vi "Simple DAQ.vi"() -> ()   [LabVIEW 2014]
uses:
  Classes/DAQ/DAQ Parameters.ctl
  Classes/DAQ/Trigger Source.ctl
  Classes/DAQ/Trigger Slope.ctl
  Type Defs/OCT DAQ Channel Data Type.ctl
  Classes/DAQ/Clock Control.ctl
  Simple DAQ States.ctl
  Classes/DAQ Control Functional Global States.ctl
  Classes/DAQ/ATS660/ATS660 Class.lvclass
  Classes/DAQ/ATS9462/ATS9462 Class.lvclass
  Classes/DAQ/ATS9350/ATS9350.lvclass
  Classes/Laser/Insite/Insight.lvclass
  <vilib>/Analysis/4window.llb/Hanning Window (DBL).vi
  <vilib>/Analysis/2dsp.llb/Real FFT.vi
  <vilib>/Analysis/4window.llb/AllCosWindow (DBL).vi
  Classes/DAQ/DAQ Class.lvclass
  <vilib>/Analysis/NI_AALPro.lvlib
panel:
  out "Path append":string="\\Insight LASER\\"
  in  "Record Data":bool
  in  "LASER Source":enum16{"INSIGHT", "SANTEC"}(ring)
  out "offset":dbl format="%.2f"
  out "mult":dbl
  in  "FFT Display":bool
  out "Frequency Domain":dbl[][](graph)
  in  "Pause Button":bool
  in  "Stop Button":bool
  in  "Play Button":bool
  out "Time Domain":dbl[][](graph)
  in  "DAQ Parameters Out":T1={"Points Per A-Scan"=1024, "A-Scans Per B-Scan"=250, "Number of B-Scans"=1, "A-Scans Per Transfer"=250, "Trigger Voltage"=200.0, "Trigger Source"=enum."External", "Trigger Slope"=enum."Rising", "Channel"=enum."Channel 1", "Clock"=enum."External Clock", "Bits per Sample"=16.0, "Range"=2.0}
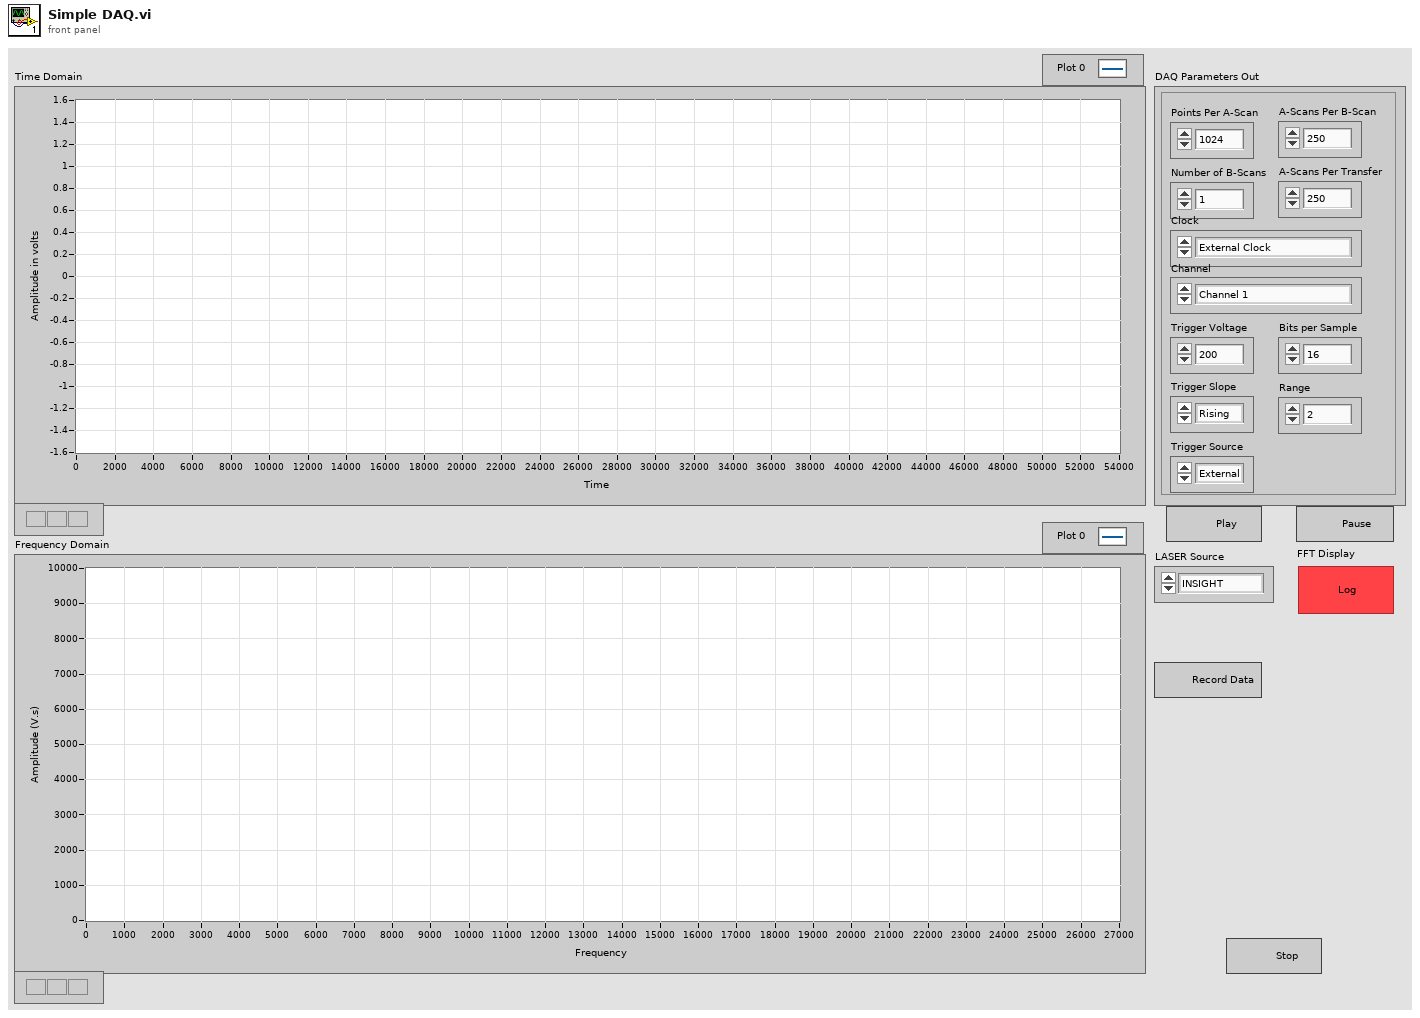
[diagram p1: front panel]
types:
  T1 = typedef "DAQ Class.lvclass/DAQ Parameters.ctl" = cluster{"Points Per A-Scan":u32, "A-Scans Per B-Scan":u32, "Number of B-Scans":u32, "A-Scans Per Transfer":u32, "Trigger Voltage":sgl, "Trigger Source":T2, "Trigger Slope":T3, "Channel":T4, "Clock":T5, "Bits per Sample":dbl, "Range":dbl}
  T2 = typedef "DAQ Class.lvclass/Trigger Source.ctl" = enum16{"External", "Channel A", "Channel B"}
  T3 = typedef "DAQ Class.lvclass/Trigger Slope.ctl" = enum16{"Rising", "Falling"}
  T4 = typedef "OCT DAQ Channel Data Type.ctl" = enum16{"Channel 1", "Channel 2", "Channel 1 and 2"}
  T5 = typedef "DAQ Class.lvclass/Clock Control.ctl" = enum16{"Internal Clock", "External Clock"}
  T6 = typedef "Simple DAQ States.ctl" = enum16{"Initialize DAQ", "Reset DAQ", "Configure DAQ", "Acquire", "Acquire and Save", "Stop"}
  T7 = typedef "DAQ Control Functional Global States.ctl" = enum16{"Status", "Set Processing Finished", "Reset", "Clear", "Set DAQ Finished"}
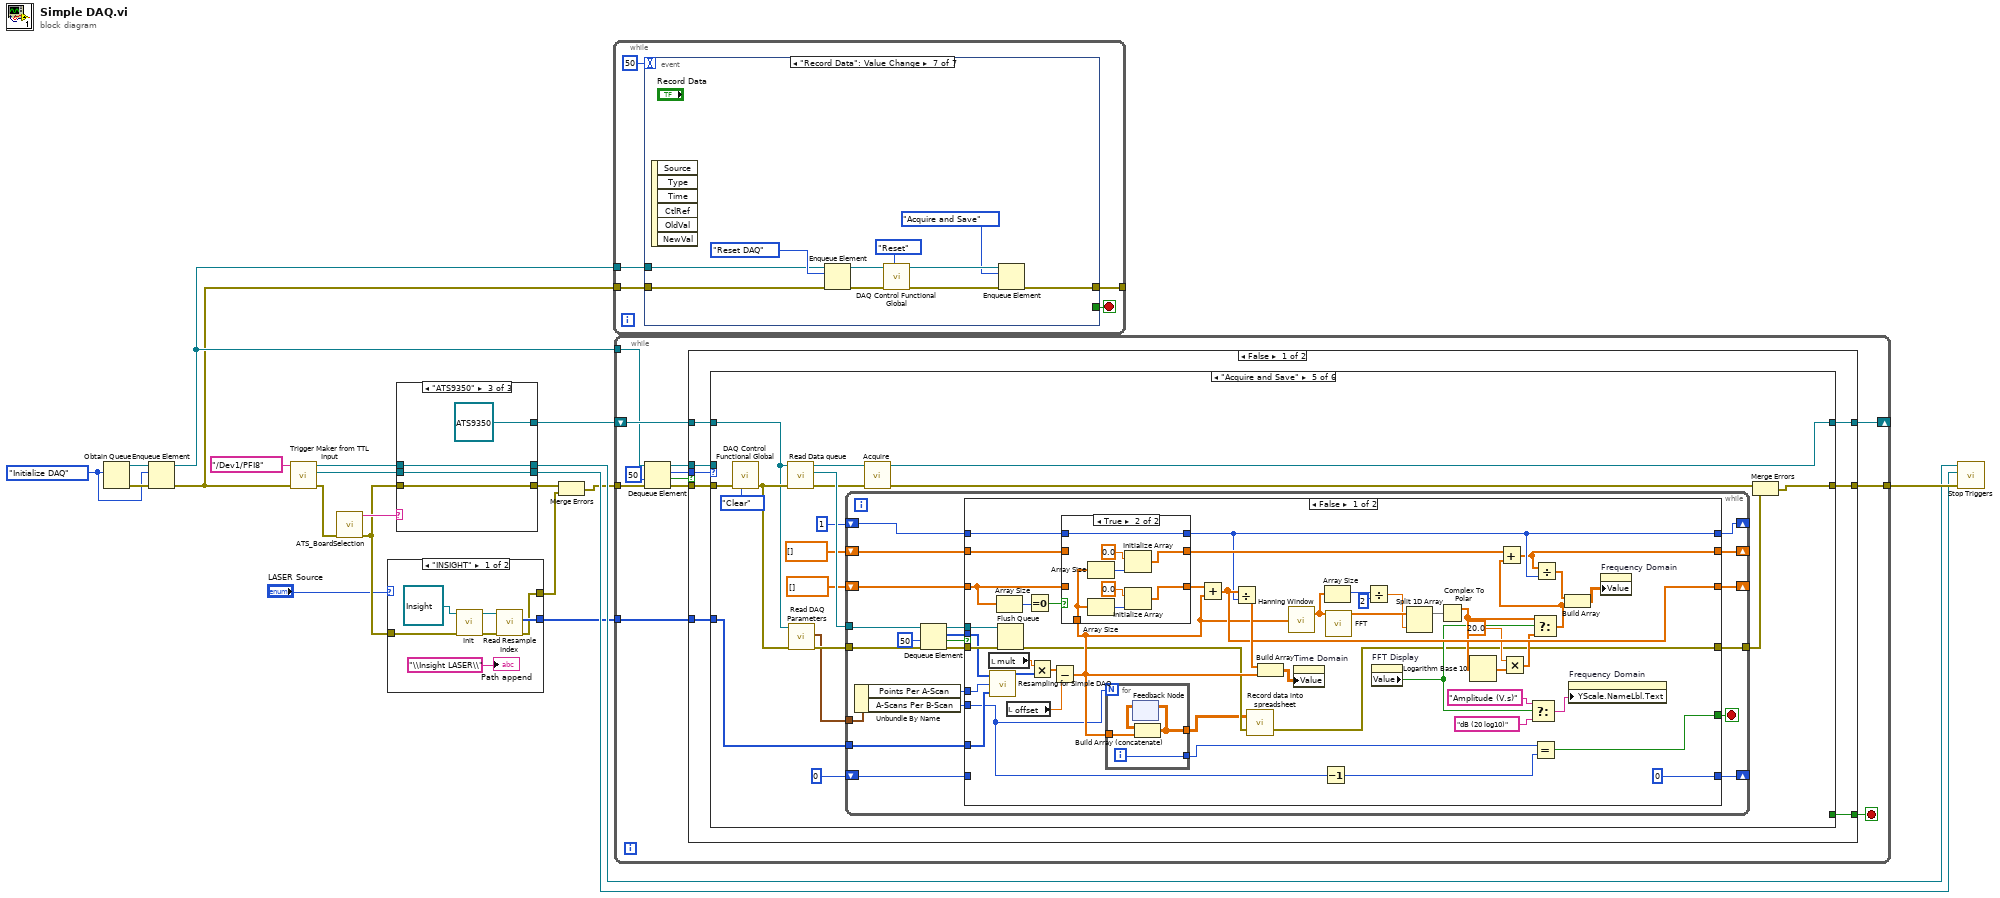
[diagram p0: block diagram]
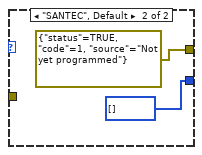
[diagram p2: hidden frame]
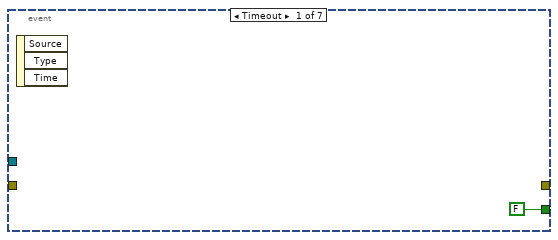
[diagram p3: hidden frame]
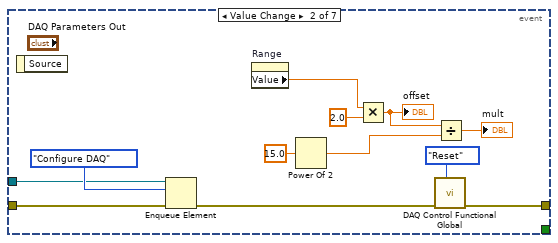
[diagram p4: hidden frame]
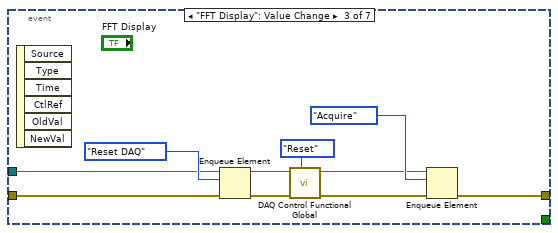
[diagram p5: hidden frame]
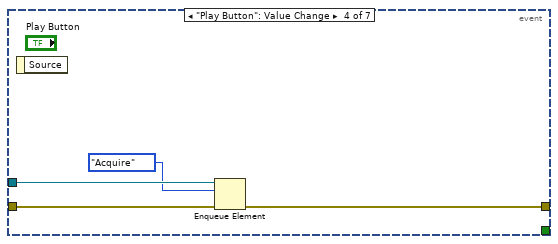
[diagram p6: hidden frame]
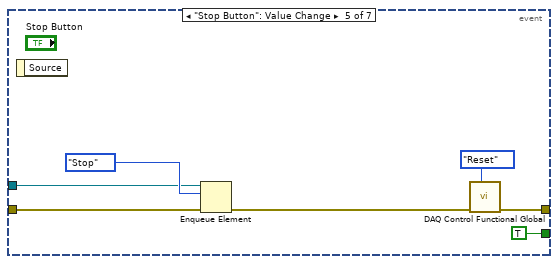
[diagram p7: hidden frame]
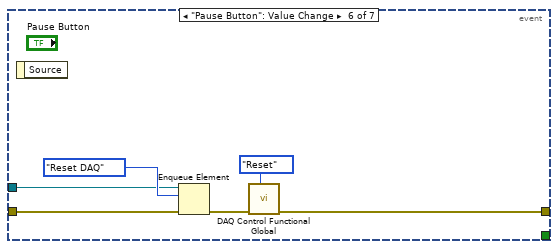
[diagram p8: hidden frame]
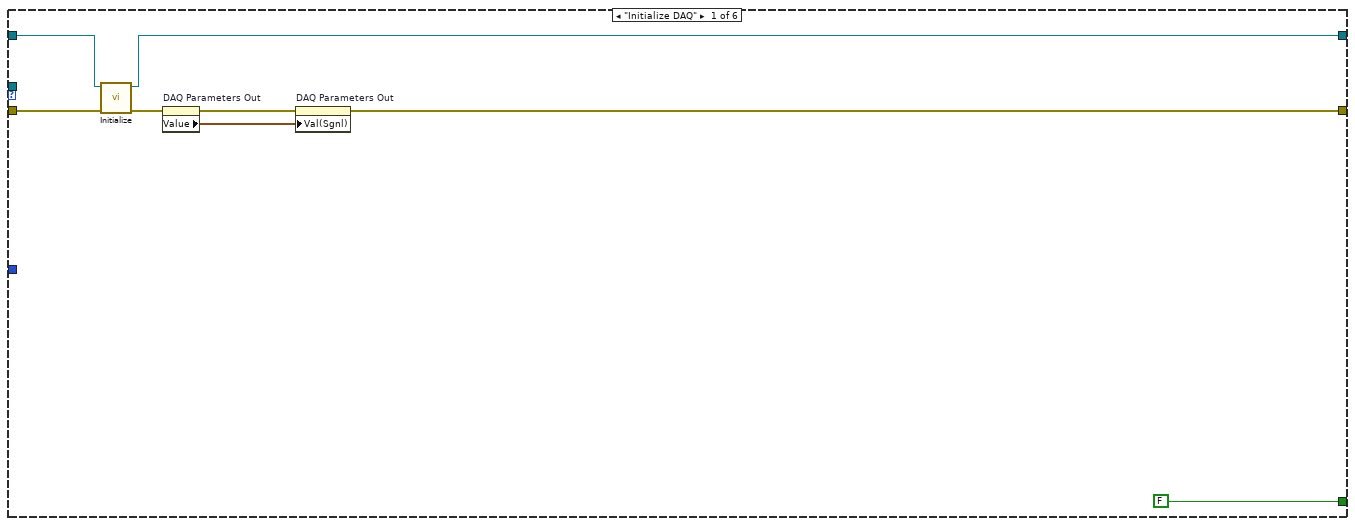
[diagram p9: hidden frame]
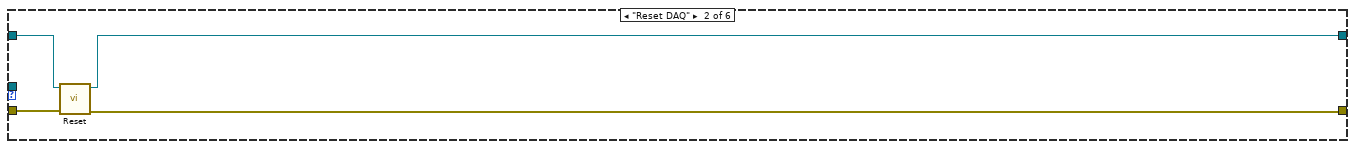
[diagram p10: hidden frame]
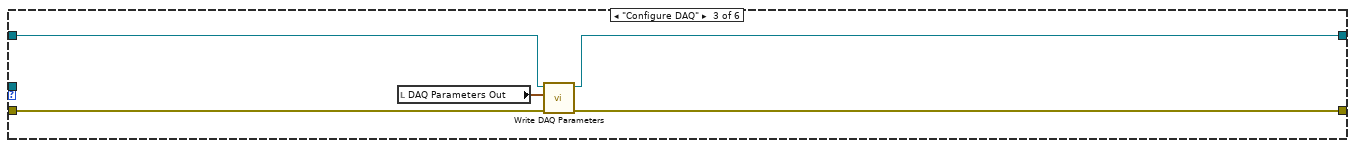
[diagram p11: hidden frame]
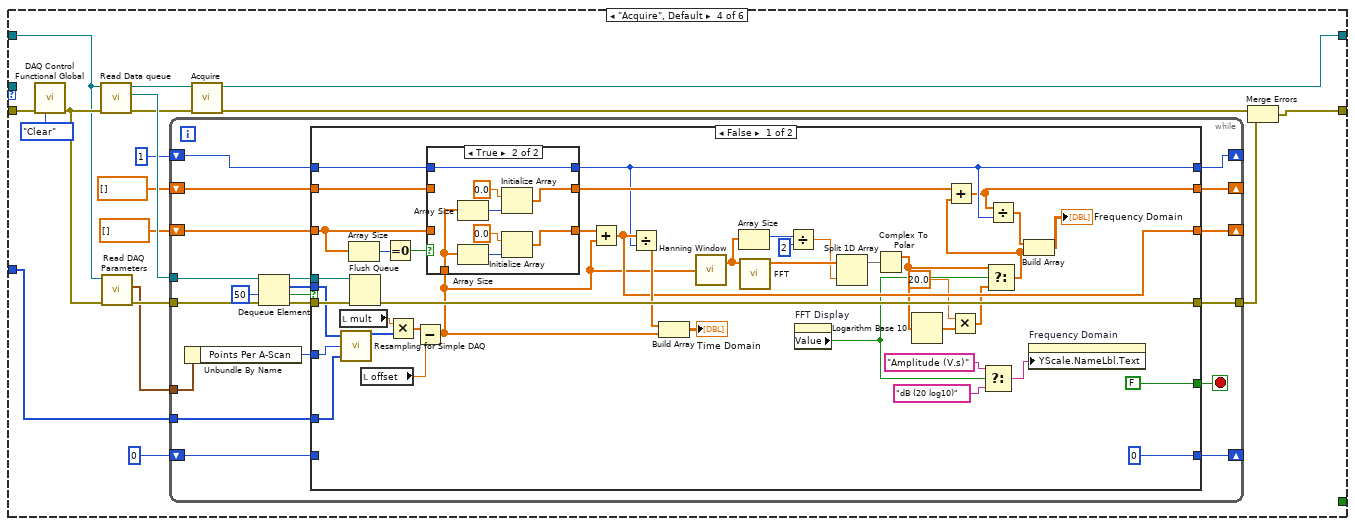
[diagram p12: hidden frame]
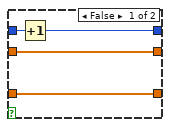
[diagram p13: hidden frame]
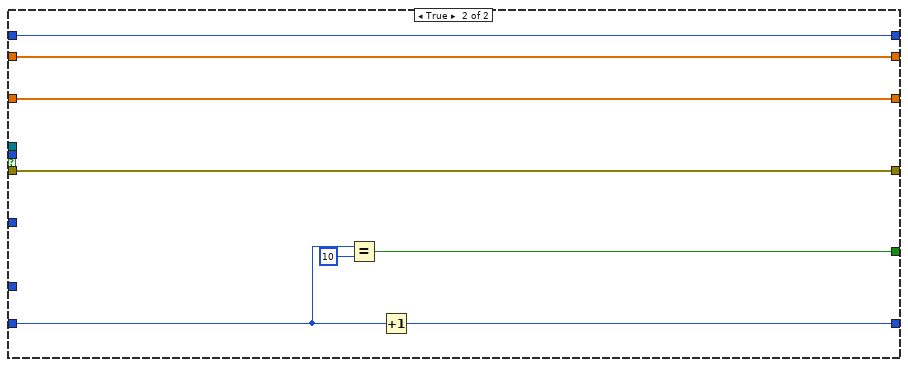
[diagram p14: hidden frame]
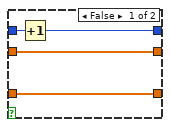
[diagram p15: hidden frame]
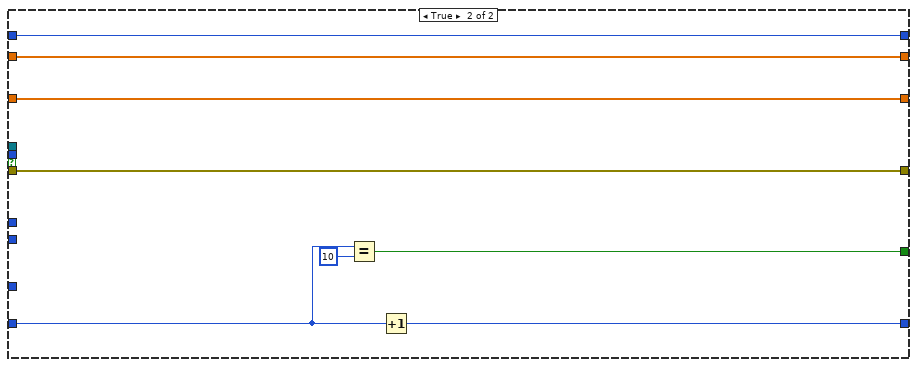
[diagram p16: hidden frame]
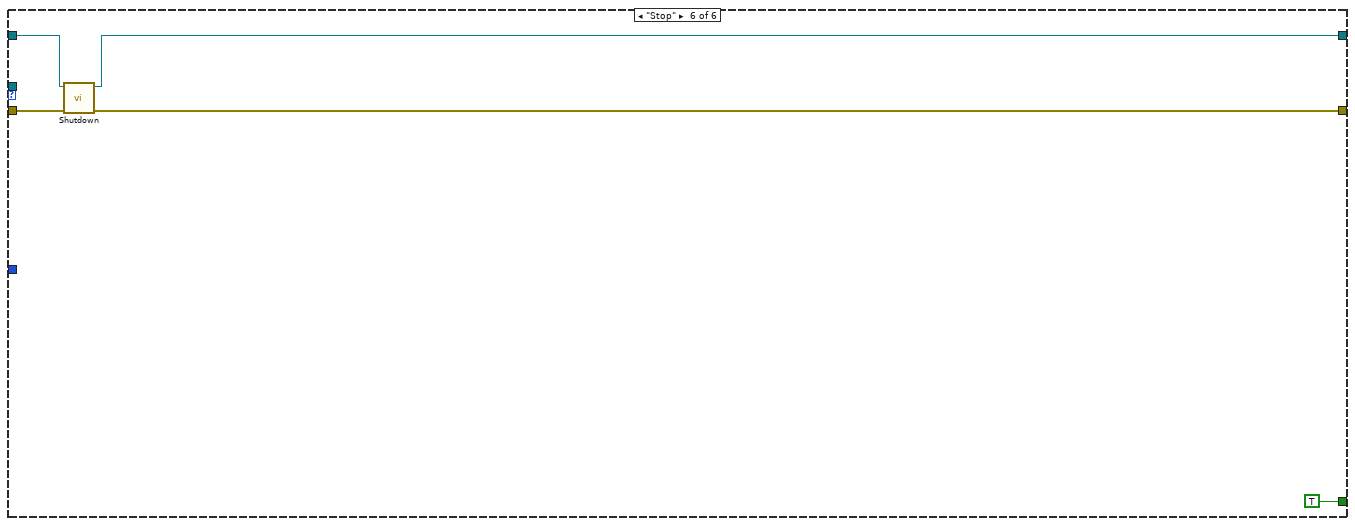
[diagram p17: hidden frame]
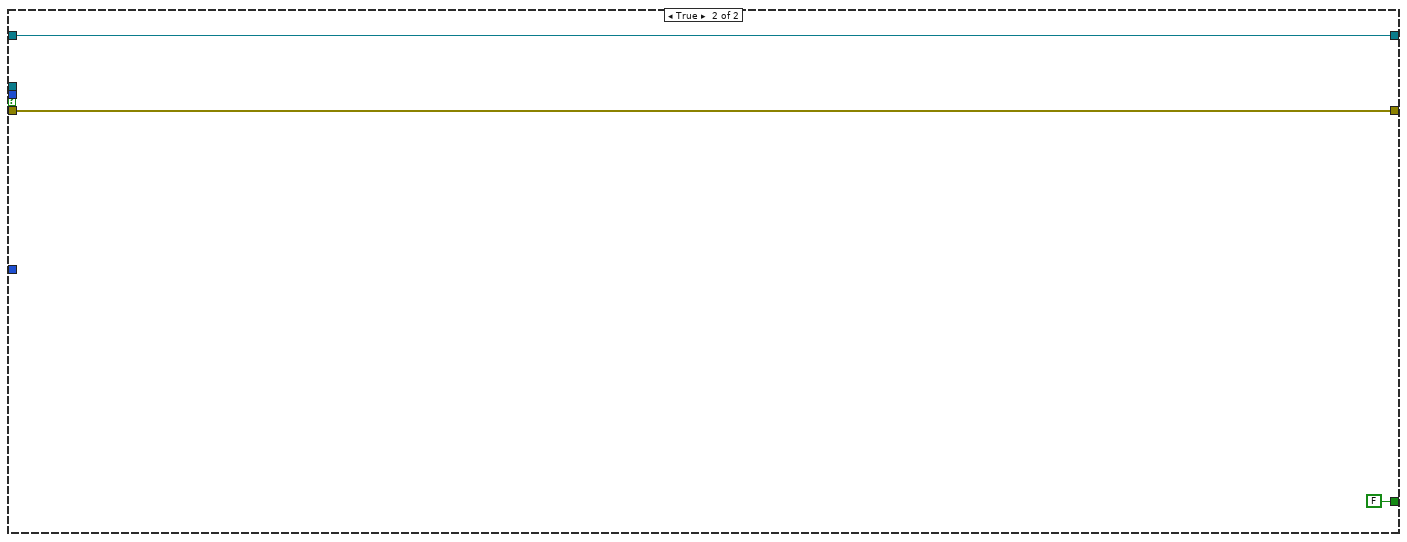
[diagram p18: hidden frame]
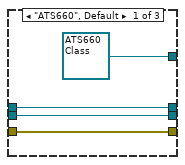
[diagram p19: hidden frame]
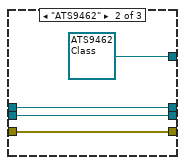
[diagram p20: hidden frame]
diagram:
  w8 = Simple_DAQ_States."Initialize DAQ" ("Simple OCT States")
  n1 = Obtain Queue(element data type=w8) -> (queue out=w12:refnum<queue>, error out=w11:errorcluster)  [unwired: 4 in, 1 out]
  n2 = Enqueue Element(queue=w12, element=w8, error in (no error)=w11) -> (queue out=w10:refnum<queue>, error out=w9:errorcluster)  [unwired: 1 in, 1 out]
  n3 = call "Trigger Maker from TTL Input.vi"("Error in"=w9, "Master Trigger In from Laser (TTL)"=tag "/Dev1/PFI8") -> ("error out"=w7:errorcluster, "Alazar Task"=w18:refnum<k21>, "AFG11000 Task"=w19:refnum<k21>)  [unwired: 7 in]
  n4 = call "ATS_BoardSelection.vi"("error in (no error)"=w7) -> ("error out"=w5:errorcluster, "Board"=w6:string)  [unwired: 9 in]
  n5 = case shown="\"INSIGHT\"" "LASER Source" {
    tunnel: w5 -> [w21 _]
    tunnel: [w27 u32[] [] ("Resample Index")] -> w3
    tunnel: [w26 errorcluster {"status"=TRUE, "code"=1, "source"="Not yet programmed"} ("error constant")] -> w1
    frame "INSIGHT" {
      n6 = call-dynamic "Init.vi"("error in (no error)"=w21, "Insite in"=refnum<class "Insight.lvclass"> refnum ("Insight.lvclass")) -> ("error out"=w22:errorcluster, "Insite out"=w23:refnum<class "Insight.lvclass">)  [unwired: 8 in]
      n7 = call-dynamic "Read Resample Index.vi"("error in (no error)"=w22, "Laser in"=w23) -> ("error out"=w26:errorcluster, "Resample Index"=w27:u32[])  [unwired: 7 in, 1 out]
      "Path append" <- "\\Insight LASER\\"
    }
    frame "SANTEC", Default {
    }
  }
  n8 = case shown="\"ATS9350\"" w6 {
    tunnel: w5 -> [w31 w34 w39]
    tunnel: [w33 w36 w41] -> w14
    tunnel: w19 -> [w33 w36 w41]
    tunnel: w18 -> [w32 w35 w40]
    tunnel: [w32 w35 w40] -> w13
    tunnel: [w31 w34 w39] -> w17
    tunnel: [refnum<class "ATS660 Class.lvclass"> refnum ("ATS660 Class.lvclass") refnum<class "ATS9462 Class.lvclass"> refnum ("ATS9462 Class.lvclass") refnum<class "ATS9350.lvclass"> refnum ("ATS9350.lvclass")] -> w16
    frame "ATS660", Default {
    }
    frame "ATS9462" {
    }
    frame "ATS9350" {
    }
  }
  n9 = Merge Errors(w17, w1) -> (w2:errorcluster)
  n10 = while {
    tunnel: w10 -> [w43]
    tunnel: w9 -> [w44]
    tunnel: [w42] -> _
    stop <- w46 stop-if-true
    n11 = event shown="[6] \"Record Data\": Value Change" {
      selector: _ -> [_ _ _ _ _ _ _]
      dyn-events: _ -> [_ _ _ _ _ _ _]
      timeout: 50 -> [_ _ _ _ _ _ _]
      tunnel: [FALSE _ _ _ TRUE _ _] -> w46
      tunnel: w44 -> [_ w56 w64 w71 w74 w84 w87]
      tunnel: w43 -> [_ w57 w65 w72 w73 w83 w88]
      tunnel: [_ w54 w62 w70 w75 w80 w86] -> w42
      event Timeout {
        n12 = event-data() -> ()  [unwired: 1 in, 3 out]
      }
      event Value Change {
        n13 = event-data() -> ()  [unwired: 1 in, 1 out]
        n14 = Enqueue Element(queue=w57, element=Simple_DAQ_States."Configure DAQ" ("Simple OCT States"), error in (no error)=w56) -> (error out=w55:errorcluster)  [unwired: 1 in, 2 out]
        n15 = property on="Range" class="DigNum (strict)"() -> ("Value"=w49:dbl)  [unwired: 2 in, 2 out]
        n16 = Power Of 2(x=15.0) -> (2^x=w52:dbl)
        n17 = Multiply(x=w49, y=2.0 ("Offset")) -> (x*y=w48:dbl)
        "offset" <- w48
        n18 = call "DAQ Control Functional Global.vi"("State"=DAQ_Control_Functional_Global_States."Reset", "Error In"=w55) -> ("Error Out"=w54:errorcluster)  [unwired: 6 in, 3 out]
        n19 = Divide(x=w48, y=w52) -> (x/y=→"mult":dbl)
      }
      event "FFT Display": Value Change {
        n20 = event-data() -> ()  [unwired: 1 in, 6 out]
        n21 = Enqueue Element(queue=w65, element=Simple_DAQ_States."Reset DAQ" ("Simple OCT States"), error in (no error)=w64) -> (queue out=w60:refnum<queue>, error out=w68:errorcluster)  [unwired: 1 in, 1 out]
        n22 = call "DAQ Control Functional Global.vi"("State"=DAQ_Control_Functional_Global_States."Reset", "Error In"=w68) -> ("Error Out"=w61:errorcluster)  [unwired: 6 in, 3 out]
        n23 = Enqueue Element(queue=w60, element=Simple_DAQ_States."Acquire" ("Simple OCT States"), error in (no error)=w61) -> (error out=w62:errorcluster)  [unwired: 1 in, 2 out]
      }
      event "Play Button": Value Change {
        n24 = event-data() -> ()  [unwired: 1 in, 1 out]
        n25 = Enqueue Element(queue=w72, element=Simple_DAQ_States."Acquire" ("Simple OCT States"), error in (no error)=w71) -> (error out=w70:errorcluster)  [unwired: 1 in, 2 out]
      }
      event "Stop Button": Value Change {
        n26 = event-data() -> ()  [unwired: 1 in, 1 out]
        n27 = Enqueue Element(queue=w73, element=Simple_DAQ_States."Stop" ("Simple OCT States"), error in (no error)=w74) -> (error out=w76:errorcluster)  [unwired: 1 in, 2 out]
        n28 = call "DAQ Control Functional Global.vi"("State"=DAQ_Control_Functional_Global_States."Reset", "Error In"=w76) -> ("Error Out"=w75:errorcluster)  [unwired: 6 in, 3 out]
      }
      event "Pause Button": Value Change {
        n29 = event-data() -> ()  [unwired: 1 in, 1 out]
        n30 = Enqueue Element(queue=w83, element=Simple_DAQ_States."Reset DAQ" ("Simple OCT States"), error in (no error)=w84) -> (error out=w81:errorcluster)  [unwired: 1 in, 2 out]
        n31 = call "DAQ Control Functional Global.vi"("State"=DAQ_Control_Functional_Global_States."Reset", "Error In"=w81) -> ("Error Out"=w80:errorcluster)  [unwired: 6 in, 3 out]
      }
      event "Record Data": Value Change {
        n32 = event-data() -> ()  [unwired: 1 in, 6 out]
        n33 = Enqueue Element(queue=w88, element=Simple_DAQ_States."Reset DAQ" ("Simple OCT States"), error in (no error)=w87) -> (queue out=w94:refnum<queue>, error out=w89:errorcluster)  [unwired: 1 in, 1 out]
        n34 = call "DAQ Control Functional Global.vi"("State"=DAQ_Control_Functional_Global_States."Reset", "Error In"=w89) -> ("Error Out"=w93:errorcluster)  [unwired: 6 in, 3 out]
        n35 = Enqueue Element(queue=w94, element=Simple_DAQ_States."Acquire and Save" ("Simple OCT States"), error in (no error)=w93) -> (error out=w86:errorcluster)  [unwired: 1 in, 2 out]
      }
    }
  }
  n36 = while {
    tunnel: w2 -> [w104]
    tunnel: w10 -> [w100]
    tunnel: [w97] -> w15
    shift-right: [w96] -> _
    shift-left: w16 -> [w106]
    tunnel: w3 -> [w95]
    stop <- w105 stop-if-true
    n37 = Dequeue Element(queue=w100, timeout in ms (-1)=50, error in (no error)=w104) -> (queue out=w99:refnum<queue>, element=w98:T6, timed out?=w101:bool, error out=w103:errorcluster)
    n38 = case shown="False" w101 {
      tunnel: w103 -> [w114 w349]
      tunnel: w106 -> [w113 w347]
      tunnel: [w111 FALSE] -> w105
      tunnel: w99 -> [w108 _]
      tunnel: w98 -> [w112 _]
      tunnel: [w110 w349] -> w97
      tunnel: [w109 w347] -> w96
      tunnel: w95 -> [w107 _]
      frame False {
        n39 = case shown="\"Acquire and Save\"" w112 {
          tunnel: w114 -> [w122 w126 w131 w141 w241 w346]
          tunnel: w113 -> [w121 w125 w130 w135 w235 w345]
          tunnel: [FALSE _ _ _ _ TRUE] -> w111
          tunnel: [w115 w123 w128 w139 w239 w343] -> w110
          tunnel: [w119 w124 w127 w140 w240 w344] -> w109
          tunnel: w108 -> [_ _ _ _ _ _]
          tunnel: w107 -> [_ _ _ w132 w232 _]
          frame "Initialize DAQ" {
            n40 = call-dynamic "Initialize.vi"("error in (no error)"=w122, "DAQ Class in"=w121) -> ("error out"=w118:errorcluster, "DAQ Class out"=w119:refnum<class "DAQ Class.lvclass">)  [unwired: 8 in]
            n41 = property on="DAQ Parameters Out" class="Clust (strict)"(error in=w118) -> (error out=w117:errorcluster, "Value"=w116:T1)  [unwired: 1 in, 1 out]
            n42 = property on="DAQ Parameters Out" class="Clust (strict)"(error in=w117, "Val(Sgnl)"=w116) -> (error out=w115:errorcluster)  [unwired: 1 in, 1 out]
          }
          frame "Reset DAQ" {
            n43 = call-dynamic "Reset.vi"("error in (no error)"=w126, "DAQ Class in"=w125) -> ("error out"=w123:errorcluster, "DAQ Class out"=w124:refnum<class "DAQ Class.lvclass">)  [unwired: 8 in]
          }
          frame "Configure DAQ" {
            n44 = local read "DAQ Parameters Out"() -> (w129:T1)
            n45 = call-dynamic "Write DAQ Parameters.vi"("error in (no error)"=w131, "DAQ Parameters"=w129, "DAQ Class in"=w130) -> ("error out"=w128:errorcluster, "DAQ Class out"=w127:refnum<class "DAQ Class.lvclass">)  [unwired: 7 in]
          }
          frame "Acquire", Default {
            n46 = call "DAQ Control Functional Global.vi"("State"=DAQ_Control_Functional_Global_States."Clear", "Error In"=w141) -> ("Error Out"=w136:errorcluster)  [unwired: 6 in, 3 out]
            n47 = call-dynamic "Read Data queue.vi"("error in (no error)"=w136, "DAQ Class in"=w135) -> ("error out"=w147:errorcluster, "Data queue"=w148:refnum<queue>, "DAQ Class out"=w149:refnum<class "DAQ Class.lvclass">)  [unwired: 7 in]
            n48 = call-dynamic "Read DAQ Parameters.vi"("error in (no error)"=w136, "DAQ Class in"=w135) -> ("error out"=w137:errorcluster, "DAQ Parameters"=w134:T1)  [unwired: 7 in, 1 out]
            n49 = while {
              tunnel: w148 -> [w169]
              tunnel: w137 -> [w168]
              shift-right: [w160] -> _
              shift-left: sgl[] [] -> [w165]
              shift-right: [w158] -> _
              shift-left: 1 -> [w159]
              tunnel: [w157] -> w144
              shift-right: [w155] -> _
              shift-left: 0 -> [w156]
              tunnel: w134 -> [w154]
              shift-right: [w152] -> _
              shift-left: sgl[] [] -> [w153]
              tunnel: w132 -> [w151]
              stop <- w166 stop-if-true
              n50 = Unbundle By Name(w154) -> ("Points Per A-Scan"=w150:u32)
              n51 = Dequeue Element(queue=w169, timeout in ms (-1)=50, error in (no error)=w168) -> (queue out=w162:refnum<queue>, element=w161:u16[], timed out?=w164:bool, error out=w163:errorcluster)
              n52 = case shown="False" w164 {
                tunnel: [FALSE w225] -> w166
                tunnel: w165 -> [w207 w231]
                tunnel: w163 -> [w210 w229]
                tunnel: w162 -> [w211 _]
                tunnel: w161 -> [w201 _]
                tunnel: [w197 w231] -> w160
                tunnel: w159 -> [w205 w230]
                tunnel: [w188 w230] -> w158
                tunnel: [w204 w229] -> w157
                tunnel: w156 -> [_ w227]
                tunnel: [0 w228] -> w155
                tunnel: w150 -> [w200 _]
                tunnel: w153 -> [w196 w224]
                tunnel: [w187 w224] -> w152
                tunnel: w151 -> [w170 _]
                frame False {
                  n53 = local read "mult"() -> (w173:dbl)
                  n54 = call "Resampling for Simple DAQ.vi"("Resample Index"=w170, "Points Per A-Scan"=w200, "U16 Array"=w201) -> ("Array"=w174:u16[])
                  n55 = Array Size(array=w207) -> (size(s)=w209:i32)
                  n56 = Flush Queue(queue=w211, error in (no error)=w210) -> (error out=w204:errorcluster)  [unwired: 2 out]
                  n57 = local read "offset"() -> (w172:dbl)
                  n58 = Equal To 0?(x=w209) -> (x = 0?=w208:bool)
                  n59 = Multiply(x=w173, y=w174) -> (x*y=w175:dbl[])
                  n60 = Subtract(x=w175, y=w172) -> (x-y=w171:dbl[])
                  n61 = case shown="True" w208 {
                    tunnel: w171 -> [_ w216]
                    tunnel: w207 -> [w215 _]
                    tunnel: [w215 w221] -> w206
                    tunnel: w205 -> [w214 w220]
                    tunnel: [w213 w220] -> w188
                    tunnel: w196 -> [w212 _]
                    tunnel: [w212 w217] -> w192
                    frame False {
                      n62 = Increment(x=w214) -> (x+1=w213:i32)
                    }
                    frame True {
                      n63 = Array Size(array=w216) -> (size(s)=w218:i32)
                      n64 = Array Size(array=w216) -> (size(s)=w223:i32)
                      n65 = Initialize Array(sgl 0.0 ("element"), w218) -> (w217:sgl[])
                      n66 = Initialize Array(sgl 0.0 ("element"), w223) -> (w221:sgl[])
                    }
                  }
                  n67 = Add(x=w206, y=w171) -> (x+y=w197:dbl[])
                  n68 = Divide(x=w197, y=w188) -> (x/y=w199:dbl[])
                  n69 = Build Array(w199, w171) -> (→"Time Domain":dbl[][])
                  n70 = call-poly <vilib>:"Hanning Window.vi"("X"=w171) -> ("Windowed X"=w195:dbl[])  [unwired: 1 out]
                  n71 = Array Size(array=w195) -> (size(s)=w194:i32)
                  n72 = call-poly <vilib>:"FFT.vi"("X"=w195) -> ("FFT {X}"=w191:cdb[])  [unwired: 9 in, 1 out]
                  n73 = Divide(x=w194, y=2) -> (x/y=w190:dbl)
                  n74 = property on="FFT Display" class="Bool (strict)"() -> ("Value"=w176:bool)  [unwired: 2 in, 2 out]
                  n75 = Split 1D Array(array=w191, index=w190) -> (first subarray=w189:cdb[])  [unwired: 1 out]
                  n76 = Complex To Polar(r * e^(i*theta)=w189) -> (r=w184:dbl[])  [unwired: 1 out]
                  n77 = Logarithm Base 10(1:w184) -> (0:w183:dbl[])
                  n78 = Multiply(x=20.0, y=w183) -> (x*y=w181:dbl[])
                  n79 = Select(t="Amplitude (V.s)", s=w176, f="dB (20 log10)") -> (s? t:f=w179:string)
                  n80 = Select(t=w184, s=w176, f=w181) -> (s? t:f=w180:dbl[])
                  n81 = Add(x=w192, y=w180) -> (x+y=w187:dbl[])
                  n82 = Divide(x=w187, y=w188) -> (x/y=w185:dbl[])
                  n83 = Build Array(w185, w180) -> (→"Frequency Domain":dbl[][])
                  n84 = property on="Frequency Domain" class="WFGraph (strict)"("YScale.NameLbl.Text"=w179) -> ()  [unwired: 2 in, 2 out]
                }
                frame True {
                  n85 = Equal?(x=w227, y=10) -> (x = y?=w225:bool)
                  n86 = Increment(x=w227) -> (x+1=w228:i32)
                }
              }
            }
            n87 = call-dynamic "Acquire.vi"("error in (no error)"=w147, "DAQ Class in"=w149) -> ("error out"=w143:errorcluster, "DAQ Class out"=w140:refnum<class "DAQ Class.lvclass">)  [unwired: 8 in]
            n88 = Merge Errors(w143, w144) -> (w139:errorcluster)
          }
          frame "Acquire and Save" {
            n89 = call "DAQ Control Functional Global.vi"("State"=DAQ_Control_Functional_Global_States."Clear", "Error In"=w241) -> ("Error Out"=w236:errorcluster)  [unwired: 6 in, 3 out]
            n90 = call-dynamic "Read Data queue.vi"("error in (no error)"=w236, "DAQ Class in"=w235) -> ("error out"=w247:errorcluster, "Data queue"=w248:refnum<queue>, "DAQ Class out"=w249:refnum<class "DAQ Class.lvclass">)  [unwired: 7 in]
            n91 = call-dynamic "Read DAQ Parameters.vi"("error in (no error)"=w236, "DAQ Class in"=w235) -> ("error out"=w237:errorcluster, "DAQ Parameters"=w234:T1)  [unwired: 7 in, 1 out]
            n92 = while {
              tunnel: w248 -> [w270]
              tunnel: w237 -> [w269]
              shift-right: [w261] -> _
              shift-left: sgl[] [] -> [w266]
              shift-right: [w259] -> _
              shift-left: 1 -> [w260]
              tunnel: [w258] -> w244
              shift-right: [w256] -> _
              shift-left: 0 -> [w257]
              tunnel: w234 -> [w255]
              shift-right: [w253] -> _
              shift-left: sgl[] [] -> [w254]
              tunnel: w232 -> [w252]
              stop <- w267 stop-if-true
              n93 = Unbundle By Name(w255) -> ("Points Per A-Scan"=w251:u32, "A-Scans Per B-Scan"=w250:u32)
              n94 = Dequeue Element(queue=w270, timeout in ms (-1)=50, error in (no error)=w269) -> (queue out=w263:refnum<queue>, element=w262:u16[], timed out?=w265:bool, error out=w264:errorcluster)
              n95 = case shown="False" w265 {
                tunnel: [w272 w335] -> w267
                tunnel: w266 -> [w313 w341]
                tunnel: w264 -> [w316 w339]
                tunnel: w263 -> [w317 _]
                tunnel: w262 -> [w309 _]
                tunnel: [w306 w341] -> w261
                tunnel: w260 -> [w311 w340]
                tunnel: [w297 w340] -> w259
                tunnel: [w276 w339] -> w258
                tunnel: w257 -> [_ w337]
                tunnel: [0 w338] -> w256
                tunnel: w251 -> [w308 _]
                tunnel: w254 -> [w305 w334]
                tunnel: [w296 w334] -> w253
                tunnel: w252 -> [w281 _]
                tunnel: w250 -> [w273 _]
                frame False {
                  n96 = local read "mult"() -> (w283:dbl)
                  n97 = call "Resampling for Simple DAQ.vi"("Resample Index"=w281, "Points Per A-Scan"=w308, "U16 Array"=w309) -> ("Array"=w284:u16[])
                  n98 = Array Size(array=w313) -> (size(s)=w315:i32)
                  n99 = Flush Queue(queue=w317, error in (no error)=w316) -> (error out=w277:errorcluster)  [unwired: 2 out]
                  n100 = local read "offset"() -> (w282:dbl)
                  n101 = Equal To 0?(x=w315) -> (x = 0?=w314:bool)
                  n102 = Multiply(x=w283, y=w284) -> (x*y=w285:dbl[])
                  n103 = Subtract(x=w285, y=w282) -> (x-y=w278:dbl[])
                  n104 = case shown="True" w314 {
                    tunnel: w278 -> [_ w326]
                    tunnel: w313 -> [w325 _]
                    tunnel: [w325 w331] -> w312
                    tunnel: w311 -> [w324 w330]
                    tunnel: [w323 w330] -> w297
                    tunnel: w305 -> [w322 _]
                    tunnel: [w322 w327] -> w301
                    frame False {
                      n105 = Increment(x=w324) -> (x+1=w323:i32)
                    }
                    frame True {
                      n106 = Array Size(array=w326) -> (size(s)=w328:i32)
                      n107 = Array Size(array=w326) -> (size(s)=w333:i32)
                      n108 = Initialize Array(sgl 0.0 ("element"), w328) -> (w327:sgl[])
                      n109 = Initialize Array(sgl 0.0 ("element"), w333) -> (w331:sgl[])
                    }
                  }
                  n110 = for {
                    N: w273 -> [_]
                    tunnel: w278 -> [w321]
                    tunnel: [w319] -> w271
                    tunnel: [w318] -> w275
                    i -> [w318]
                    n111 = feedback #1() -> (w320:dbl[][])  [unwired: 1 in]
                    n112 = Build Array (concatenate)(w320, w321) -> (w319:dbl[][])
                    n113 = feedback-in #1(w319) -> ()
                  }
                  n114 = Add(x=w312, y=w278) -> (x+y=w306:dbl[])
                  n115 = Divide(x=w306, y=w297) -> (x/y=w307:dbl[])
                  n116 = call "Record data into spreadsheet.vi"("Error In"=w277, "Data"=w271) -> ("Error Out"=w276:errorcluster)  [unwired: 1 in]
                  n117 = Build Array(w307, w278) -> (w279:dbl[][])
                  n118 = call-poly <vilib>:"Hanning Window.vi"("X"=w278) -> ("Windowed X"=w304:dbl[])  [unwired: 1 out]
                  n119 = property on="Time Domain" class="WFGraph (strict)"("Value"=w279) -> ()  [unwired: 2 in, 2 out]
                  n120 = Decrement(x=w273) -> (x-1=w274:u32)
                  n121 = Array Size(array=w304) -> (size(s)=w303:i32)
                  n122 = call-poly <vilib>:"FFT.vi"("X"=w304) -> ("FFT {X}"=w300:cdb[])  [unwired: 9 in, 1 out]
                  n123 = Divide(x=w303, y=2) -> (x/y=w299:dbl)
                  n124 = property on="FFT Display" class="Bool (strict)"() -> ("Value"=w286:bool)  [unwired: 2 in, 2 out]
                  n125 = Split 1D Array(array=w300, index=w299) -> (first subarray=w298:cdb[])  [unwired: 1 out]
                  n126 = Complex To Polar(r * e^(i*theta)=w298) -> (r=w294:dbl[])  [unwired: 1 out]
                  n127 = Logarithm Base 10(1:w294) -> (0:w293:dbl[])
                  n128 = Multiply(x=20.0, y=w293) -> (x*y=w291:dbl[])
                  n129 = Select(t="Amplitude (V.s)", s=w286, f="dB (20 log10)") -> (s? t:f=w289:string)
                  n130 = Select(t=w294, s=w286, f=w291) -> (s? t:f=w290:dbl[])
                  n131 = Add(x=w301, y=w290) -> (x+y=w296:dbl[])
                  n132 = Equal?(x=w275, y=w274) -> (x = y?=w272:bool)
                  n133 = Divide(x=w296, y=w297) -> (x/y=w295:dbl[])
                  n134 = Build Array(w295, w290) -> (w280:dbl[][])
                  n135 = property on="Frequency Domain" class="WFGraph (strict)"("YScale.NameLbl.Text"=w289) -> ()  [unwired: 2 in, 2 out]
                  n136 = property on="Frequency Domain" class="WFGraph (strict)"("Value"=w280) -> ()  [unwired: 2 in, 2 out]
                }
                frame True {
                  n137 = Equal?(x=w337, y=10) -> (x = y?=w335:bool)
                  n138 = Increment(x=w337) -> (x+1=w338:i32)
                }
              }
            }
            n139 = call-dynamic "Acquire.vi"("error in (no error)"=w247, "DAQ Class in"=w249) -> ("error out"=w243:errorcluster, "DAQ Class out"=w240:refnum<class "DAQ Class.lvclass">)  [unwired: 8 in]
            n140 = Merge Errors(w243, w244) -> (w239:errorcluster)
          }
          frame "Stop" {
            n141 = call-dynamic "Shutdown.vi"("error in (no error)"=w346, "DAQ Class in"=w345) -> ("error out"=w343:errorcluster, "DAQ Class out"=w344:refnum<class "DAQ Class.lvclass">)  [unwired: 8 in]
          }
        }
      }
      frame True {
      }
    }
  }
  n142 = call "Stop Triggers.vi"("Error in"=w15, "Alazar Task"=w13, "AFG11000 Task"=w14) -> ()  [unwired: 8 in, 1 out]
